vi "write channel limits from RT config file.vi"(10 "configFileRef":T3, 11 "RT config":T19={"Message"={"Parameters"={"FPGA Ref"=refnum, "configID"=0, "activeChannels"=[]}, "Variables"={"RT Status"={"Comms loop"=FALSE, "scheduler loop"=FALSE, "data process loop"=FALSE, "FIFO loop"=FALSE, "Command Stream"=FALSE, "Error Stream"=FALSE, "FPGA FIFO"=FALSE, "Data Stream"=FALSE}, "watchdog"=timestamp(0 s since 1904-01-01), "limitsEnabled"=FALSE, "Interlocks"={"gearboxOil"=FALSE, "bearingOil"=FALSE, "gearboxAir"=FALSE}}}, "FIFO"={"Params"={"FPGA ref"=refnum, "Total Channels"=0}, "Variables"={"FIFO wait counter"=0, "FIFO read trigger"=0}}, "Comms data"={"Parameters"={"error writer name"="", "command reader name"="", "error buffer size"=0, "command buffer size"=0, "scanivalveIP"="", "scanivalvePeriod"=0}, "Variables"={"listen schedule"=0, "incident buffer"=[], "command stream"="", "error stream"="", "waiting for command stream connect"=FALSE, "waiting for error stream connect"=FALSE, "scanivalve connection"=refnum, "scanivalveScheduleID"=0, "activeScanivalvePorts"=[], "channelCount"=0}, "scanivalveConfig"={"listS"={"period"=0, "ADtrig"=FALSE, "ScanTrig"=FALSE, "page"=0, "qpkts"=0}, "listC"={"ZC"=FALSE, "unitScan"="", "CvtUnit"=0.0, "bin"=FALSE, "EU"=FALSE}, "listSG"={"Avg1"=0, "FPS1"=0, "SGEnable1"=FALSE}, "activeChannels"={"Chan1"={"101"=FALSE, "102"=FALSE, "103"=FALSE, "104"=FALSE, "109"=FALSE, "110"=FALSE, "111"=FALSE, "112"=FALSE, "201"=FALSE, "202"=FALSE, "203"=FALSE, "204"=FALSE, "209"=FALSE, "210"=FALSE, "211"=FALSE, "212"=FALSE, "301"=FALSE, "302"=FALSE, "303"=FALSE, "304"=FALSE, "309"=FALSE, "310"=FALSE, "311"=FALSE, "312"=FALSE, "401"=FALSE, "402"=FALSE, "403"=FALSE, "404"=FALSE, "409"=FALSE, "410"=FALSE, "411"=FALSE, "412"=FALSE}}}}, "Data processor"={"Parameters"={"FPGA Ref"=refnum, "data stream"={"data writer name"="error writer", "NS write buffer size"=16, "NS Buffer length"=0}, "FIFO Depth"=0, "Channel controls"={"FIFO channel count"=0, "active indices"=[], "active channels"=0, "channelScaling"=[], "scanivalveCount"=0, "channels"=[]}, "safetyChannels"={"oilP"=0, "airP"=0, "water"=0, "channelLimits"=[]}, "speedChannel"=0, "maxSpeedLimit"=0.0, "Torque"={"fixedOffset"=0.0, "filter"=FALSE, "fallingEdge"=FALSE, "swapEncoders"=FALSE}}, "Variables"={"Intermediary buffer"=[], "buffer position"=0, "write loop counter"=0, "NS write trigger"=0, "NS Connection status"=FALSE, "waiting for NS"=FALSE, "labAmbient"={"pressure"=0.0, "temperature"=0.0}, "scanivalvePorts"=[], "scanivalvePressures"=[], "data stream"="", "activeChannelLimitIndex"=[], "runningSpeedLimit"=0.0, "speedChannelIndex"=0, "Interlocks"={"gearboxOil"=FALSE, "bearingOil"=FALSE, "gearboxAir"=FALSE}, "interlockChannels"={"gearboxOil"=0, "bearingOil"=0, "air"=0}, "limitStates"=[]}}}) -> ()   [LabVIEW 2018]
uses:
  RT/Type Defs/Message loop data.ctl
  RT/Type Defs/FPGA reference.ctl
  RT/Type Defs/RT Status.ctl
  RT/Type Defs/Analogue loop data.ctl
  RT/Communications loop/comms data.ctl
  RT/Type Defs/generic incident.ctl
  ICL-LabVIEW_General/Scanivalve API project/full interface/polymorphic/scanivalveConfig.ctl
  ICL-LabVIEW_General/Scanivalve API project/full interface/listS.ctl
  ICL-LabVIEW_General/Scanivalve API project/full interface/listC.ctl
  ICL-LabVIEW_General/Scanivalve API project/full interface/listSG.ctl
  ICL-LabVIEW_General/Scanivalve API project/full interface/chan1.ctl
  RT/Type Defs/Data processing loop data.ctl
  type defs/channelControl.ctl
  RT/Type Defs/channelScalingTypes.ctl
  RT/Type Defs/scalingMethods.ctl
  ICL-LabVIEW_General/data channels/parent class/Data Channel.lvclass
  type defs/channelLimitControl.ctl
  type defs/limitActions.ctl
  <vilib>/Utility/config.llb/Config Data RefNum.ctl
  <vilib>/Utility/config.llb/Write Key (U32).vi
  <vilib>/Utility/config.llb/Write Key (Boolean).vi
  <vilib>/Utility/config.llb/Write Key (Double).vi
  <vilib>/Utility/config.llb/Write Key (I32).vi
  <vilib>/Utility/config.llb/NI_LVConfig.lvlib
  ICL-LabVIEW_General/Scanivalve API project/Scanivalve API.lvlib
panel:
  out "removed limits":string[](array[string])
  out "Data processor.Parameters.safetyChannels.temperatures":T1[](array[typedef])
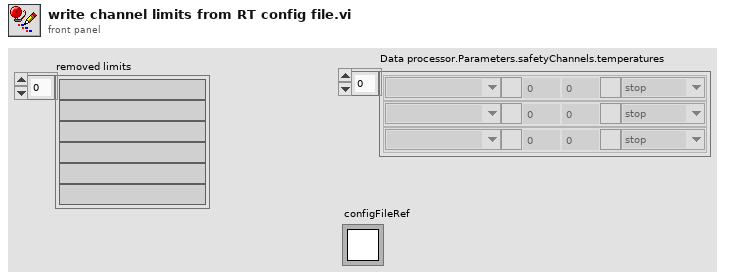
[diagram p1: front panel]
types:
  T1 = typedef "channelLimitControl.ctl" = cluster{"channelID":u16, "Enabled":bool, "warnValue":dbl, "limitValue":dbl, "Invert":bool, "limitAction":T2}
  T2 = typedef "limitActions.ctl" = enum16{"stop", "shutdown", "ignore"}
  T3 = typedef "NI_LVConfig.lvlib/Config Data RefNum.ctl" = refnum<k1>
  T4 = typedef "Message loop data.ctl" = cluster{"Parameters":cluster{"FPGA Ref":T5, "configID":u32, "activeChannels":cluster{"index":u16, "name":string}[]}, "Variables":cluster{"RT Status":T6, "watchdog":timestamp, "limitsEnabled":bool, "Interlocks":cluster{"gearboxOil":bool, "bearingOil":bool, "gearboxAir":bool}}}
  T5 = typedef "FPGA reference.ctl" = refnum<k20>
  T6 = typedef "RT Status.ctl" = cluster{"Comms loop":bool, "scheduler loop":bool, "data process loop":bool, "FIFO loop":bool, "Command Stream":bool, "Error Stream":bool, "FPGA FIFO":bool, "Data Stream":bool}
  T7 = typedef "Analogue loop data.ctl" = cluster{"Params":cluster{"FPGA ref":T5, "Total Channels":u32}, "Variables":cluster{"FIFO wait counter":u16, "FIFO read trigger":u32}}
  T8 = typedef "comms data.ctl" = cluster{"Parameters":cluster{"error writer name":string, "command reader name":string, "error buffer size":i32, "command buffer size":i32, "scanivalveIP":string, "scanivalvePeriod":u16}, "Variables":cluster{"listen schedule":u32, "incident buffer":T9[], "command stream":refnum<k21>, "error stream":refnum<k21>, "waiting for command stream connect":bool, "waiting for error stream connect":bool, "scanivalve connection":refnum<k5>, "scanivalveScheduleID":u32, "activeScanivalvePorts":i32[], "channelCount":i16}, "scanivalveConfig":T10}
  T9 = typedef "generic incident.ctl" = cluster{"timestamp":timestamp, "type":string, "Variant":variant}
  T10 = typedef "Scanivalve API.lvlib/scanivalveConfig.ctl" = cluster{"listS":T11, "listC":T12, "listSG":T13, "activeChannels":T14}
  T11 = typedef "Scanivalve API.lvlib/listS.ctl" = cluster{"period":u16, "ADtrig":bool, "ScanTrig":bool, "page":u16, "qpkts":u16}
  T12 = typedef "Scanivalve API.lvlib/listC.ctl" = cluster{"ZC":bool, "unitScan":string, "CvtUnit":dbl, "bin":bool, "EU":bool}
  T13 = typedef "Scanivalve API.lvlib/listSG.ctl" = cluster{"Avg1":u16, "FPS1":u16, "SGEnable1":bool}
  T14 = typedef "Scanivalve API.lvlib/chan1.ctl" = cluster{"Chan1":cluster{"101":bool, "102":bool, "103":bool, "104":bool, "109":bool, "110":bool, "111":bool, "112":bool, "201":bool, "202":bool, "203":bool, "204":bool, "209":bool, "210":bool, "211":bool, "212":bool, "301":bool, "302":bool, "303":bool, "304":bool, "309":bool, "310":bool, "311":bool, "312":bool, "401":bool, "402":bool, "403":bool, "404":bool, "409":bool, "410":bool, "411":bool, "412":bool}}
  T15 = typedef "Data processing loop data.ctl" = cluster{"Parameters":cluster{"FPGA Ref":T5, "data stream":cluster{"data writer name":string, "NS write buffer size":i32, "NS Buffer length":u32}, "FIFO Depth":u32, "Channel controls":cluster{"FIFO channel count":i32, "active indices":i16[], "active channels":i32, "channelScaling":T16[], "scanivalveCount":i32, "channels":refnum<class "Data Channel.lvclass">[]}, "safetyChannels":cluster{"oilP":u16, "airP":u16, "water":u16, "channelLimits":T1[]}, "speedChannel":i32, "maxSpeedLimit":dbl, "Torque":cluster{"fixedOffset":dbl, "filter":bool, "fallingEdge":bool, "swapEncoders":bool}}, "Variables":cluster{"Intermediary buffer":dbl[][], "buffer position":u32, "write loop counter":u16, "NS write trigger":u32, "NS Connection status":bool, "waiting for NS":bool, "labAmbient":cluster{"pressure":dbl, "temperature":dbl}, "scanivalvePorts":u16[], "scanivalvePressures":dbl[], "data stream":refnum<k21>, "activeChannelLimitIndex":u16[], "runningSpeedLimit":dbl, "speedChannelIndex":i32, "Interlocks":cluster{"gearboxOil":bool, "bearingOil":bool, "gearboxAir":bool}, "interlockChannels":cluster{"gearboxOil":i32, "bearingOil":i32, "air":i32}, "limitStates":cluster{"warn":bool, "alarm":bool}[]}}
  T16 = typedef "channelControl.ctl" = cluster{"index":u16, "active":bool, "channelType":T17, "module":u16, "terminal":u16, "channelName":string, "scalingMethod":T18, "scalingParameters":dbl[], "scaledUnits":string, "tempOffset":dbl}
  T17 = typedef "channelScalingTypes.ctl" = enum16{"calculation", "measurement", "scanivalve", "output", "digital"}
  T18 = typedef "scalingMethods.ctl" = enum16{"none", "linear", "thermocouple", "polynomial", "encoder", "RTD"}
  T19 = cluster{"Message":T4, "FIFO":T7, "Comms data":T8, "Data processor":T15}
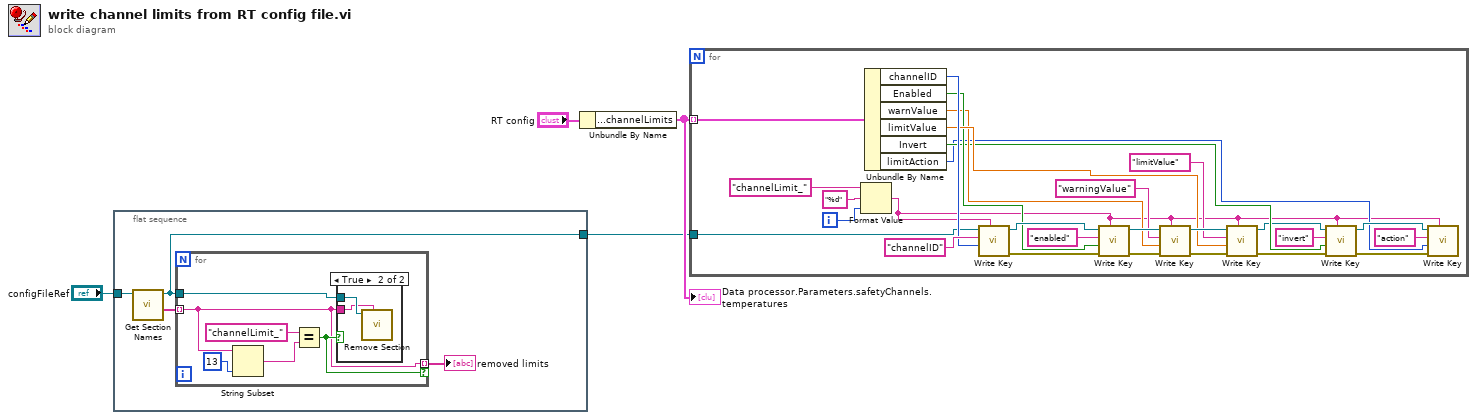
[diagram p0: block diagram]
diagram:
  n1 = flat-sequence {
    tunnel: "configFileRef" -> [w8]
    tunnel: [w5] -> w1
    frame #0 {
      n2 = call <vilib>:"Get Section Names.vi"("refnum"=w8) -> ("section names"=w7:string[], "refnum out"=w5:T3)  [unwired: 8 in, 1 out]
      n3 = for {
        tunnel: w7 -> [w9] mode=indexing
        tunnel: [w9] -> w6 mode=indexing if=w11
        tunnel: w5 -> [w10]
        n4 = String Subset(string=w9, length (rest)=13 ("length (rest)")) -> (substring=w12:string)  [unwired: 1 in]
        n5 = Equal?(x="channelLimit_" ("string (\"\")"), y=w12) -> (x = y?=w11:bool)
        n6 = case shown="True" w11 {
          tunnel: w10 -> [_ w16]
          tunnel: w9 -> [_ w15]
          frame False {
          }
          frame True {
            n7 = call <vilib>:"Remove Section.vi"("section"=w15, "refnum"=w16) -> ()  [unwired: 7 in, 3 out]
          }
        }
      }
      "removed limits" <- w6
    }
  }
  n8 = Unbundle By Name("RT config") -> ("Data processor.Parameters.safetyChannels.channelLimits"=w3:T1[])
  "Data processor.Parameters.safetyChannels.temperatures" <- w3
  n9 = for {
    tunnel: w3 -> [w41] mode=indexing
    tunnel: w1 -> [w17]
    i -> [w44]
    n10 = Format Value(string ("")="channelLimit_", format string="%d", value (0)=w44) -> (output string=w18:string)
    n11 = Unbundle By Name(w41) -> ("channelID"=w39:u16, "Enabled"=w28:bool, "warnValue"=w27:dbl, "limitValue"=w29:dbl, "Invert"=w26:bool, "limitAction"=w20:T2)
    n12 = call-poly <vilib>:"Write Key.vi"("section"=w18, "value"=w39, "key"="channelID", "refnum"=w17) -> ("error out"=w38:errorcluster, "refnum out"=w37:T3)  [unwired: 5 in, 1 out]
    n13 = call-poly <vilib>:"Write Key.vi"("section"=w18, "error in (no error)"=w38, "value"=w28, "key"="enabled", "refnum"=w37) -> ("error out"=w35:errorcluster, "refnum out"=w34:T3)  [unwired: 4 in, 1 out]
    n14 = call-poly <vilib>:"Write Key.vi"("section"=w18, "error in (no error)"=w35, "value"=w27, "key"="warningValue", "refnum"=w34) -> ("error out"=w30:errorcluster, "refnum out"=w32:T3)  [unwired: 4 in, 1 out]
    n15 = call-poly <vilib>:"Write Key.vi"("section"=w18, "error in (no error)"=w30, "value"=w29, "key"="limitValue", "refnum"=w32) -> ("error out"=w25:errorcluster, "refnum out"=w24:T3)  [unwired: 4 in, 1 out]
    n16 = call-poly <vilib>:"Write Key.vi"("section"=w18, "error in (no error)"=w25, "value"=w26, "key"="invert", "refnum"=w24) -> ("error out"=w22:errorcluster, "refnum out"=w21:T3)  [unwired: 4 in, 1 out]
    n17 = call-poly <vilib>:"Write Key.vi"("section"=w18, "error in (no error)"=w22, "value"=w20, "key"="action", "refnum"=w21) -> ()  [unwired: 4 in, 3 out]
  }
